vi "CRC Start Bit.vi"(8 "error in (no error)":errorcluster, 11 "Frame Infos":T1 {"CRC Index" min=-7 max=7; "DLC Length  Corruption Index" min=-8 max=8}) -> (0 "error out":errorcluster, 3 "CRC Start Bit":u32)   [LabVIEW 2018, in "CAN Gateway Engine.lvlib"]
uses:
  CAN Gateway Engine.lvlib
  Shared/CTLs/Frame.ctl
  Shared/CTLs/Signal_Data_Trigger.ctl
  <vilib>/xnet/xnet.llb/XNET Database Close (Signal).vi
  <resource>/objmgr/xnet.rc
  Shared/CAN Gateway Shared.lvlib
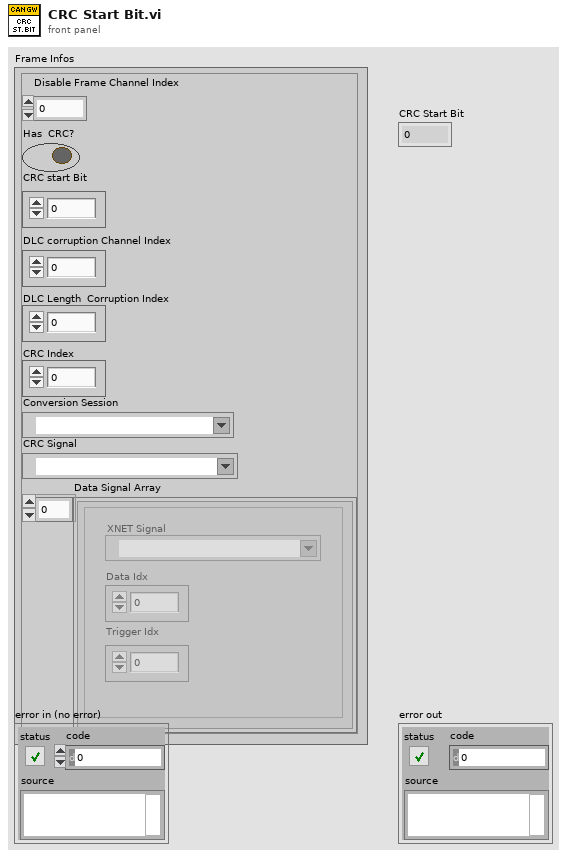
[diagram p1: front panel]
types:
  T1 = typedef "CAN Gateway Shared.lvlib/Frame.ctl" = cluster{"Disable Frame Channel Index":i32, "Has  CRC?":bool, "CRC start Bit":u32, "DLC corruption Channel Index":i32, "DLC Length  Corruption Index":i32, "CRC Index":i32, "Conversion Session":refnum<k21>, "CRC Signal":refnum<k21>, "Data Signal Array":T2[]}
  T2 = typedef "CAN Gateway Shared.lvlib/Signal_Data_Trigger.ctl" = cluster{"XNET Signal":refnum<k21>, "Data Idx":u32, "Trigger Idx":u32}
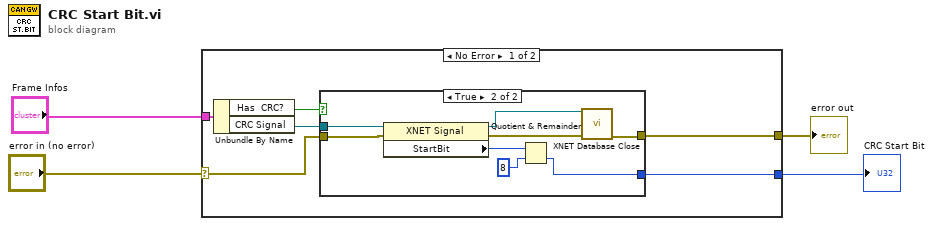
[diagram p0: block diagram]
diagram:
  n1 = case shown="No Error" "error in (no error)" {
    selector: "error in (no error)" -> [w6 w20]
    tunnel: [w10 _] -> w4
    tunnel: [w5 w20] -> w3
    tunnel: "Frame Infos" -> [w9 _]
    frame No Error {
      n2 = Unbundle By Name(w9) -> ("Has  CRC?"=w7:bool, "CRC Signal"=w8:refnum<k21>)
      n3 = case shown="True" w7 {
        tunnel: w8 -> [_ w17]
        tunnel: w6 -> [w11 w16]
        tunnel: [w11 w13] -> w5
        tunnel: [_ w12] -> w10
        frame False {
        }
        frame True {
          n4 = property class="XNET Signal"(reference=w17, error in=w16) -> (reference out=w14:refnum<k21>, error out=w15:errorcluster, "StartBit"=w19:u32)
          n5 = Quotient & Remainder(x=w19, y=u32 8) -> (floor(x/y)=w12:u32)  [unwired: 1 out]
          n6 = call-poly <vilib>:"XNET Database Close.vi"("signal in"=w14, "error in (no error)"=w15) -> ("error out"=w13:errorcluster)  [unwired: 13 in]
        }
      }
    }
    frame Error {
    }
  }
  "CRC Start Bit" <- w4
  "error out" <- w3
